vi "Update_UI_SelectedOverlay.vi"(8 "error in (no error)":errorcluster, 10 "LstBox Refnum":refnum<vi>, 11 "Image Refnum":refnum<vi>) -> (0 "error out":errorcluster)   [LabVIEW 2019]
uses:
  Controls/ROI_List_Action.ctl
  <vilib>/vision/Image Controls.llb/IMAQ Image.ctl
panel:
  in  "Vision_Image":T1(plugin-control)
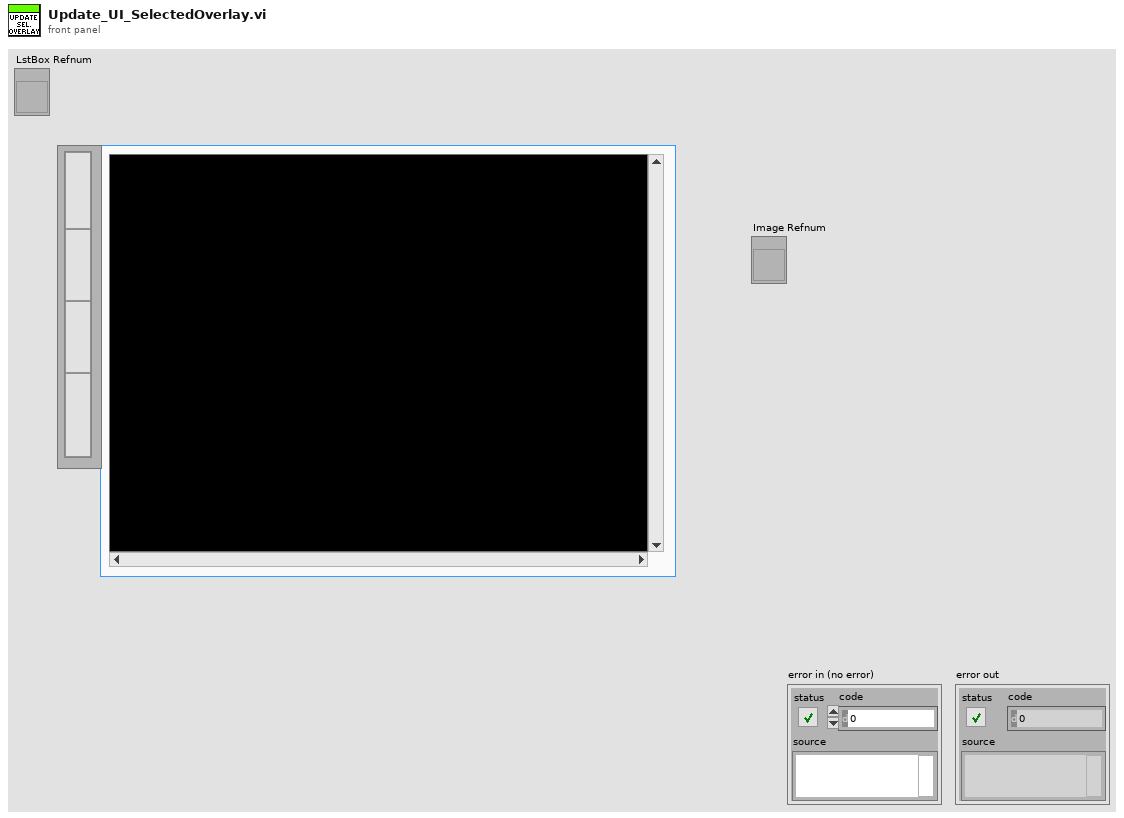
[diagram p1: front panel]
types:
  T1 = typedef "IMAQ Image.ctl" = refnum<image>
  T2 = typedef "ROI_List_Action.ctl" = enum16{"Init", "Add ROI", "Delete ROI", "Get All ROI", "Get Specific ROI", "Set Analysis Setting", "Set Process Setting", "Replace All Entries", "ROIEntryBackup", "ROIEntryBackupClear", "ROIEntryReturn"}
  T3 = typedef "Vision_DataEntry.ctl" = cluster{"vROIName":string, "vROIContour":cluster{"Contour Type":u32, "ROI Type":u32, "Points":i32[]}, "ProcessSetting":T4[], "Analysis_Setting":T6}
  T4 = typedef "Process_Setting.ctl" = cluster{"Enum_PreProcess":T5, "Parameter":string}
  T5 = typedef "VisionProcessName.ctl" = enum16{"*CamParameter*", "CamAttributes", "*Preprocess*", "CG_Brightness", "C_Plane Extraction", "C_Threshold", "G_Lookup Table", "G_Threshold"}
  T6 = typedef "Analysis_Setting.ctl" = cluster{"PreProcess":T7, "Parameter":string}
  T7 = typedef "V_Analysis_Type.ctl" = enum16{"None", "C_Color Pattern Matching", "G_PatternMatching", "G_ShapeDectect", "G_GeometricMatch", "B_Area Check"}
  T8 = cluster{"Points[0]":i32, "Points[1]":i32, "Points[2]":i32, "Points[3]":i32}
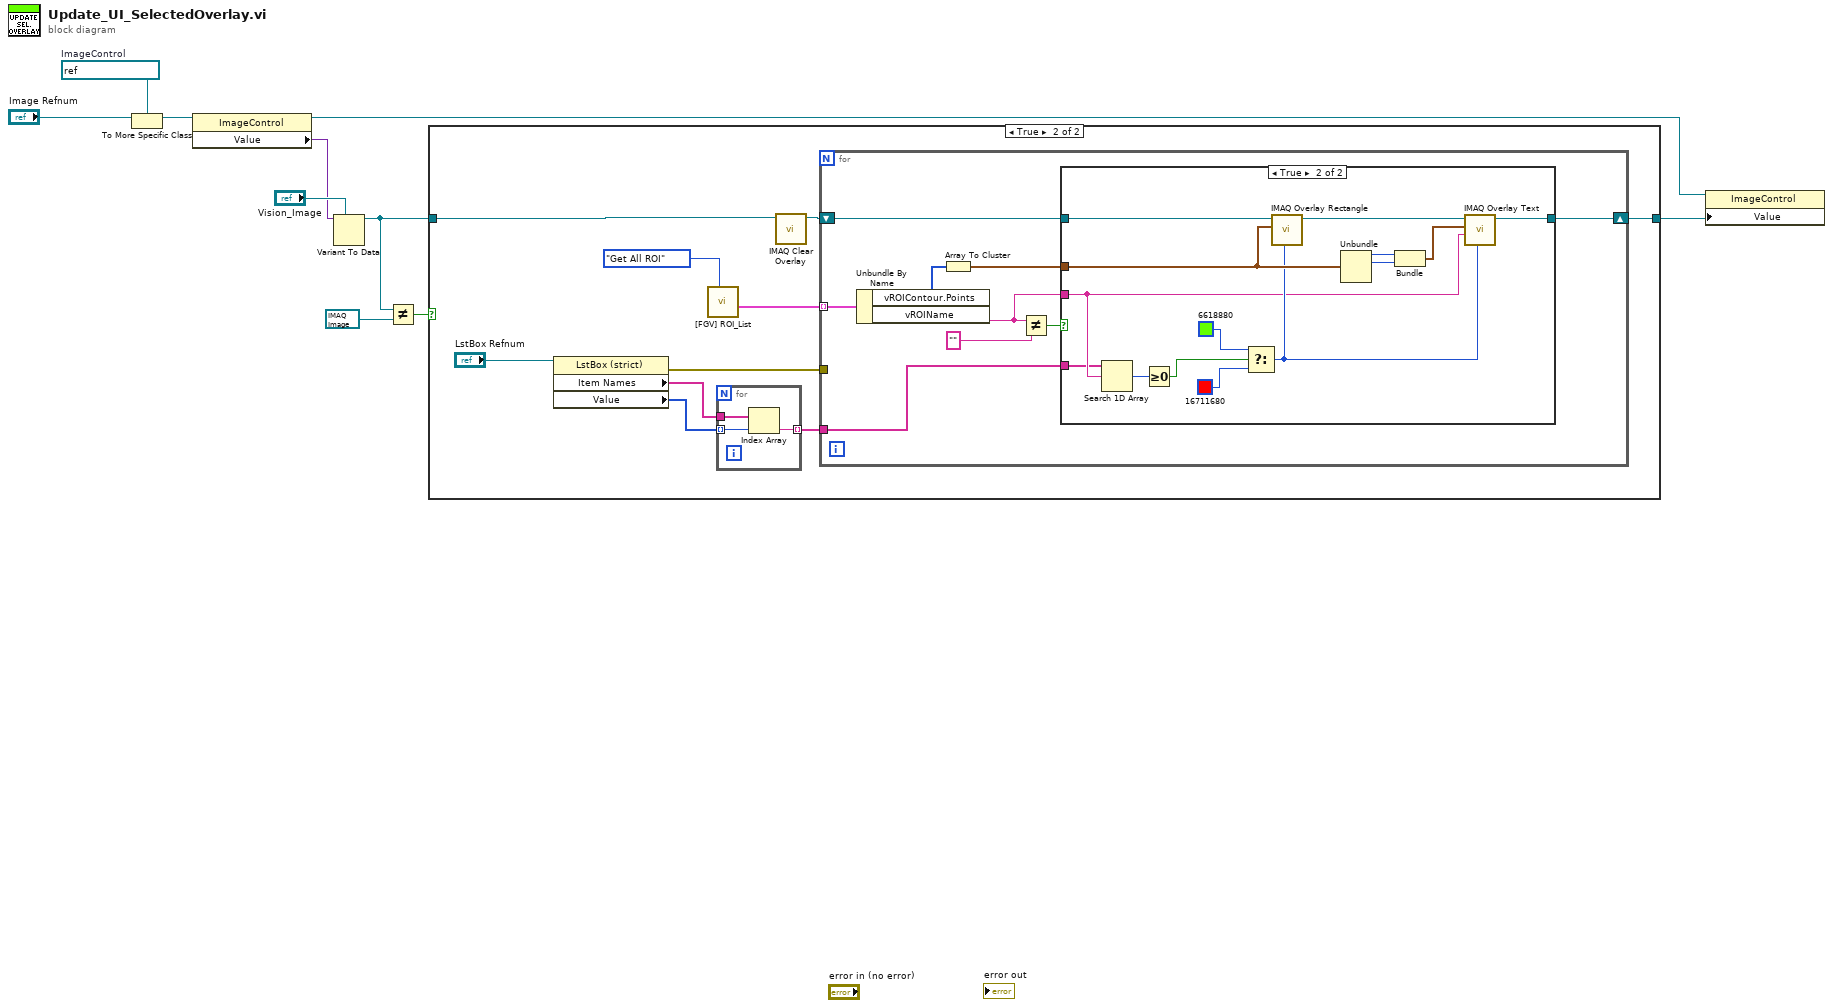
[diagram p0: block diagram]
diagram:
  w9 = refnum<vi> refnum  # ImageControl
  n1 = To More Specific Class(target class=w9, reference="Image Refnum") -> (specific class reference=w4:refnum<vi>)  [unwired: 1 in, 1 out]
  n2 = property class="ImageControl"(reference=w4) -> (reference out=w6:refnum<vi>, "Value"=w7:variant)  [unwired: 1 in, 1 out]
  n3 = Variant To Data(type="Vision_Image", Variant=w7) -> (data=w1:T1)  [unwired: 1 in, 1 out]
  n4 = Not Equal?(x=w1, y=T1 refnum ("Image Out")) -> (x != y?=w2:bool)
  n5 = case shown="True" w2 {
    tunnel: w1 -> [w11 w20]
    tunnel: [w11 w16] -> w5
    frame False {
    }
    frame True {
      n6 = property class="LstBox (strict)"(reference="LstBox Refnum") -> (error out=w15:errorcluster, "Item Names"=w13:string[], "Value"=w14:i32[])  [unwired: 1 in, 1 out]
      n7 = call "[FGV] ROI_List.vi"("Action"=ROI_List_Action."Get All ROI") -> ("All ROI"=w17:T3[])  [unwired: 8 in, 2 out]
      n8 = for {
        tunnel: w14 -> [w24] mode=indexing
        tunnel: w13 -> [w23]
        tunnel: [w22] -> w12 mode=indexing
        n9 = Index Array(array=w23, index=w24) -> (element=w22:string)
      }
      n10 = call "IMAQ Clear Overlay"("Image"=w20) -> ("Image Out"=w19:T1)  [unwired: 9 in, 1 out]
      n11 = for {
        tunnel: w17 -> [w31] mode=indexing
        shift-right: [w32] -> w16
        shift-left: w19 -> [w33]
        tunnel: w15 -> [_]
        tunnel: w12 -> [w25]
        n12 = Unbundle By Name(w31) -> ("vROIContour.Points"=w28:i32[], "vROIName"=w26:string)
        n13 = Array To Cluster(array=w28) -> (cluster=w27:T8)
        n14 = Not Equal?(x=w26, y="") -> (x != y?=w29:bool)
        n15 = case shown="True" w29 {
          tunnel: w33 -> [w34 w48]
          tunnel: [w34 w41] -> w32
          tunnel: w27 -> [_ w40]
          tunnel: w26 -> [_ w38]
          tunnel: w25 -> [_ w37]
          frame False {
          }
          frame True {
            n16 = Search 1D Array(1D array=w37, element=w38) -> (index of element=w36:i32)  [unwired: 1 in]
            n17 = Greater Or Equal To 0?(x=w36) -> (x >= 0?=w35:bool)
            n18 = Select(t=u32 6618880 ("Color"), s=w35, f=u32 16711680 ("Color")) -> (s? t:f=w39:u32)
            n19 = call "IMAQ Overlay Rectangle"("Color"=w39, "Rectangle"=w40, "Image"=w48) -> ("Image Out"=w42:T1)  [unwired: 7 in, 1 out]
            n20 = Unbundle(w40) -> ("Points[0]"=w45:i32, "Points[1]"=w44:i32)  [unwired: 2 out]
            n21 = Bundle("Points[0]"=w45, "Points[1]"=w44) -> (w43:cluster{"Points[0]":i32, "Points[1]":i32})  [unwired: 1 in]
            n22 = call "IMAQ Overlay Text"("Text Color (black)"=w39, "String"=w38, "Origin"=w43, "Image"=w42) -> ("Image Out"=w41:T1)  [unwired: 6 in, 1 out]
          }
        }
      }
    }
  }
  n23 = property class="ImageControl"(reference=w6, "Value"=w5) -> ()  [unwired: 1 in, 2 out]
